vi "Shutdown.vi"(8 "Error In":errorcluster, 11 "Parser In":refnum<class "Parser.lvclass">) -> (0 "Error Out":errorcluster, 3 "Parser Out":refnum<class "Parser.lvclass">)   [LabVIEW 2018, in "Toolkit.lvlib" / "Parser.lvclass"]
uses:
  Parser.lvclass
  Parser.lvclass/Parser.ctl
  Nodes/NonTerminal/NonTerminal.lvclass
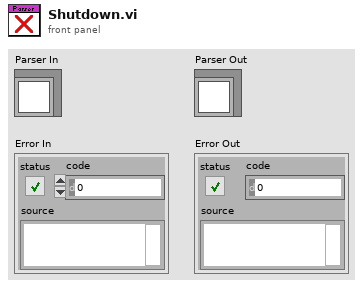
[diagram p1: front panel]
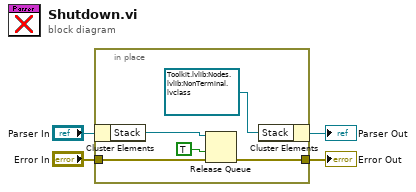
[diagram p0: block diagram]
diagram:
  n1 = in-place {
    in-place-border: "Error In" -> [w6]
    in-place-border: [w5] -> w1
    n2 = in-place-cluster #1("Parser In") -> ("Stack"=w8:refnum<queue>)
    n3 = Release Queue(queue=w8, force destroy? (F)=TRUE, error in (no error)=w6) -> (error out=w5:errorcluster)  [unwired: 2 out]
    n4 = in-place-cluster #1("Stack"=refnum<queue> refnum ("Nodes")) -> (→"Parser Out":refnum<class "Parser.lvclass">)
  }
  "Error Out" <- w1
